vi "XY Sample Stage.vi"(7 "Calling VI Ref":refnum<vi>) -> ()   [LabVIEW 2020]
uses:
  <vilib>/Utility/miscctls.llb/LVPointTypeDef.ctl
  XY Sample Stage Controls/XY Sample Stage History Actions.ctl
  XY Sample Stage Controls/XY Sample Stage XY Settings.ctl
  Hardware Configuration/Hardware Configuration Controls/Device Function.ctl
  Hardware Configuration/Hardware Configuration Controls/Device Type.ctl
  Device Library/Stages/Stages Controls/Stage Actions.ctl
panel:
  in  "Main Tabs":enum32{"XY Control", "Settings"}(tab)
  in  "Remove Current":bool
  in  "Update Current":bool
  in  "Up":bool
  in  "Halt":bool
  in  "Down":bool
  in  "Left":bool
  in  "Right":bool
  in  "Home":bool
  in  "Mark Point":bool
  in  "Clear Points":bool
  in  "Marked Positions":i32(listbox)
  out "Position History":cluster{dbl[], dbl[]}[](graph)
  in  "X Position (µm)":dbl format="%#.6f"
  in  "Y Position (µm)":dbl format="%#.6f"
  in  "Step Size (µm)":dbl format="%#.3g"
  in  "Step 1":bool
  in  "Step 2":bool
  in  "Step 3":bool
  in  "Step 4":bool
  in  "Step 5":bool
  in  "Step 6":bool
  in  "Step 7":bool
  in  "Step 8":bool
  in  "Reset Location History":bool
  in  "Active Stage":i32(ring) items=["ASI-Stage-Sample XY-COM4", "Prior-Stage-Sample Z-0.1", "Thorlabs-Stage-Adj Cavity-65864035"]
  in  "Apply Offset":bool
  in  "Flip X and Y":bool
  in  "Invert X":bool
  in  "Invert Y":bool
  in  "Save XY Config":bool
  in  "Velocity":dbl=0.17 min=0.0 max=10000.0 format="%#.6f"
  in  "X Offset":dbl min=-10000.0 max=10000.0 format="%#.6f"
  in  "Y Offset":dbl min=-10000.0 max=10000.0 format="%#.6f"
  in  "Quit":bool
  # "Preset Step Sizes"
  # "Apply Offset to Marked Positions"
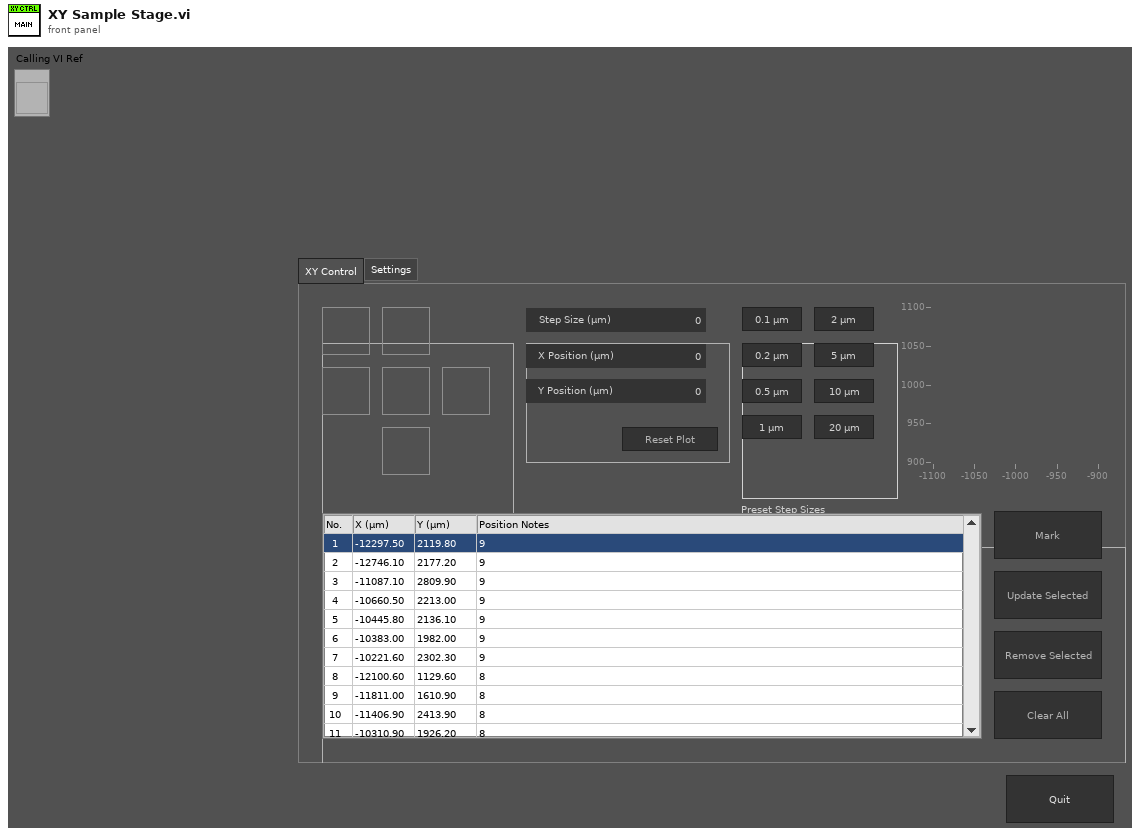
[diagram p1: front panel]
types:
  T1 = typedef "XY Sample Stage XY Settings.ctl" = cluster{"Flip X and Y":bool, "Invert X":bool, "Invert Y":bool}
  T2 = typedef "XY Sample Stage History Actions.ctl" = enum16{"Reset", "Write", "Read", "Set Zero", "Update", "Remove"}
  T3 = enum16{"Always On", "Always Off", "Off While Running"}
  T4 = typedef "LVPointTypeDef.ctl" = cluster{"Horizontal":i16, "Vertical":i16}
  T5 = typedef "LVRectTypeDef.ctl" = cluster{"Left":i16, "Top":i16, "Right":i16, "Bottom":i16}
  T6 = typedef "LVBoundsTypeDef.ctl" = cluster{"Width":u32, "Height":u32}
  T7 = typedef "Stage Actions.ctl" = enum16{"Get Position", "MVR", "MOVE", "HALT", "ONTARGET", "ERROR", "REFERENCE", "INIT", "VELOCITY", "STATUS", "EXIT", "HOME", "ZEROPOS", "NANOPOS", "ANALOG", "QUIT"}
  T8 = typedef "Device Type.ctl" = enum16{"AOTF", "Camera", "Deformable Mirror", "Laser", "Microscope Base", "Shutter", "Stage", "Waveform", "FPGA", "Email", "Filter Wheel", "Spinning Disk"}
  T9 = typedef "Device Function.ctl" = enum16{"Primary", "Secondary", "Overview", "Wide Field Drift Correction", "642 nm Excitation", "560 nm Excitation", "940 nm Excitation", "546 nm Excitation", "488 nm Excitation", "405 nm Excitation", "Objective Drift Correction", "4Pi Objective Lock", "Objective XY", "Objective Z", "Sample XY", "Sample Coarse Z", "Sample Z", "4Pi Lower", "4Pi Upper", "Mojo", "Adj Cavity", "Line Scanning", "Alert"}
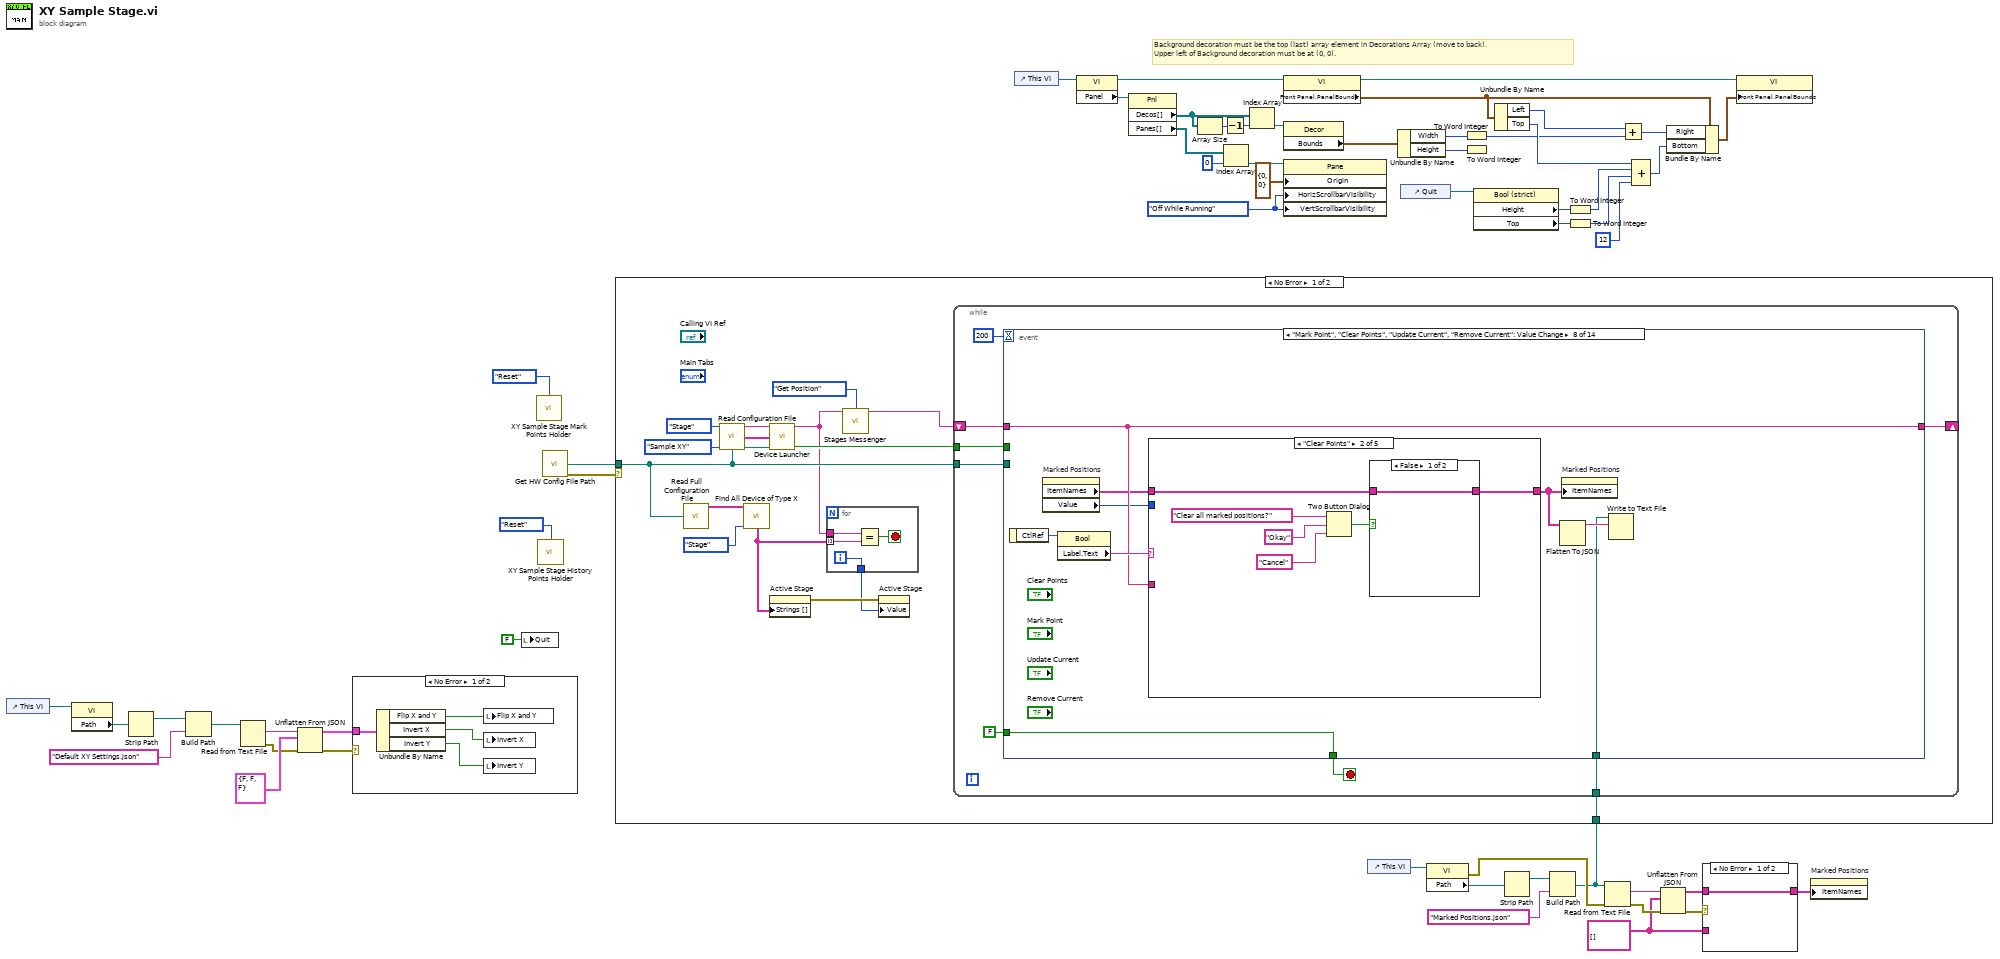
[diagram p0: block diagram]
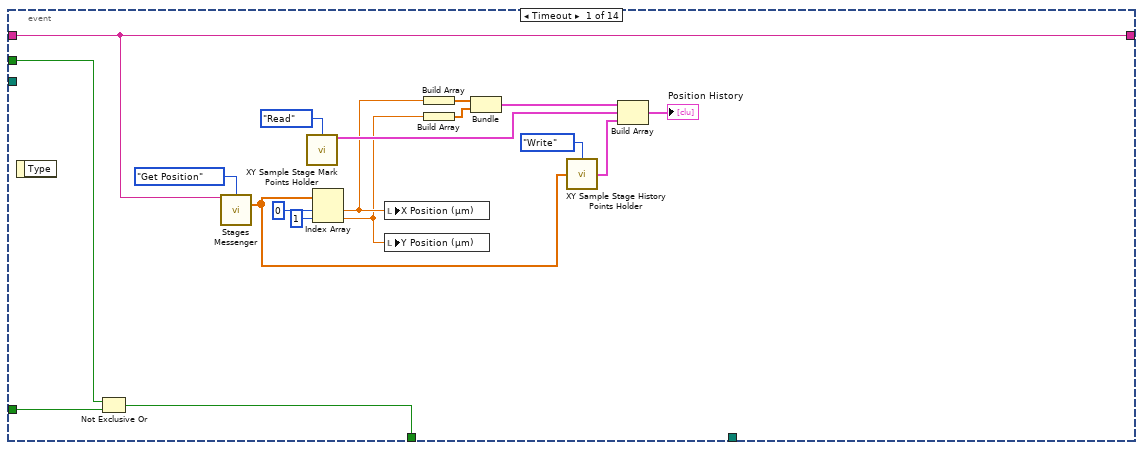
[diagram p4: hidden frame]
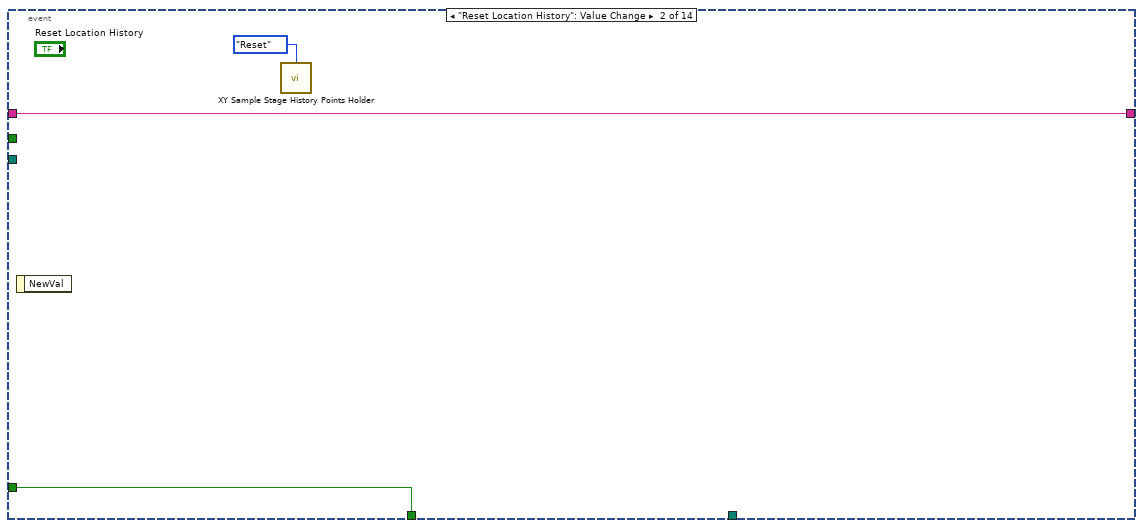
[diagram p5: hidden frame]
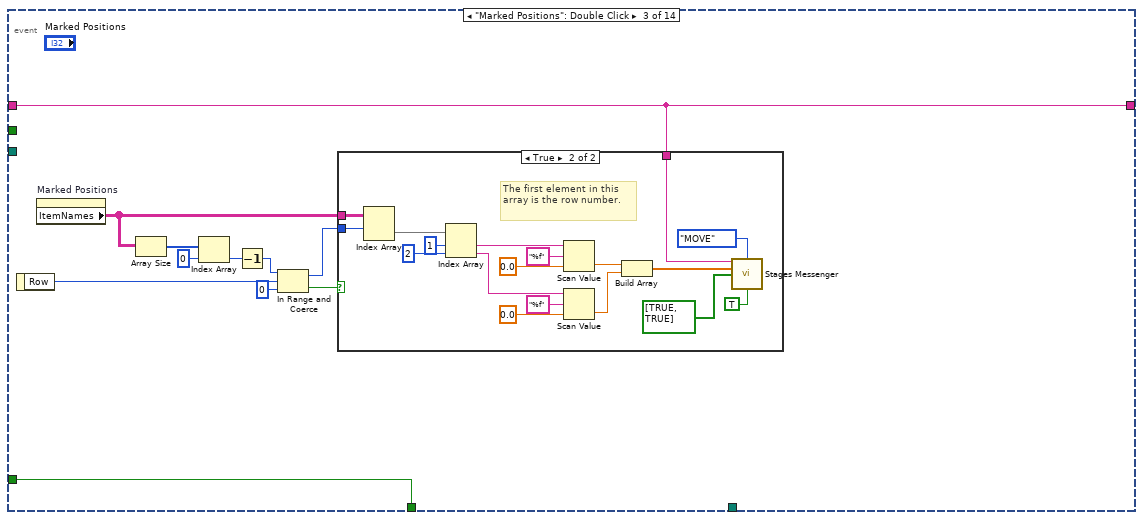
[diagram p6: hidden frame]
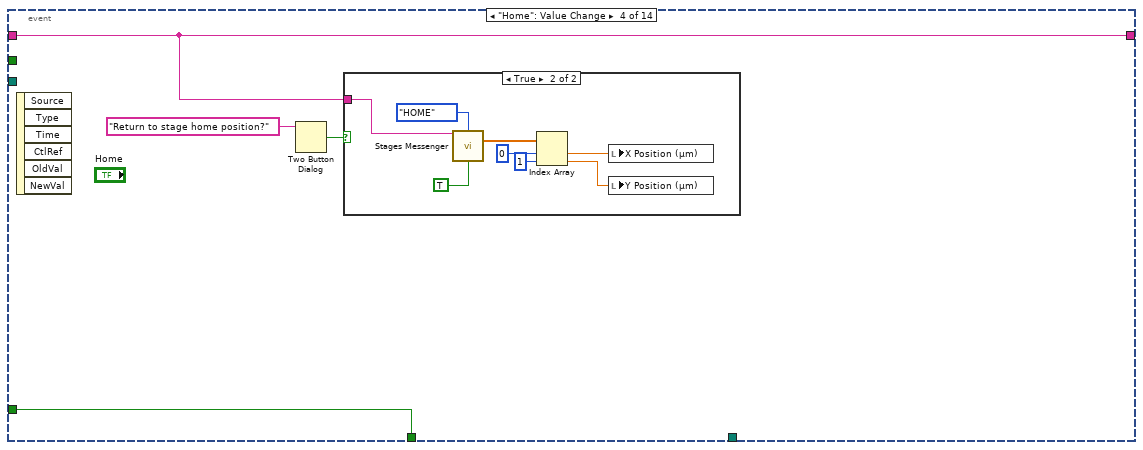
[diagram p8: hidden frame]
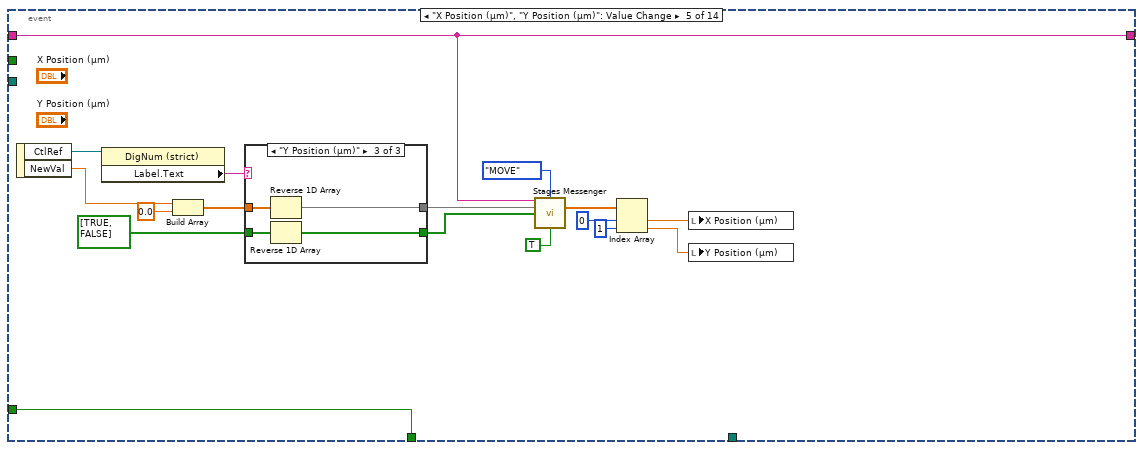
[diagram p10: hidden frame]
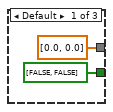
[diagram p11: hidden frame]
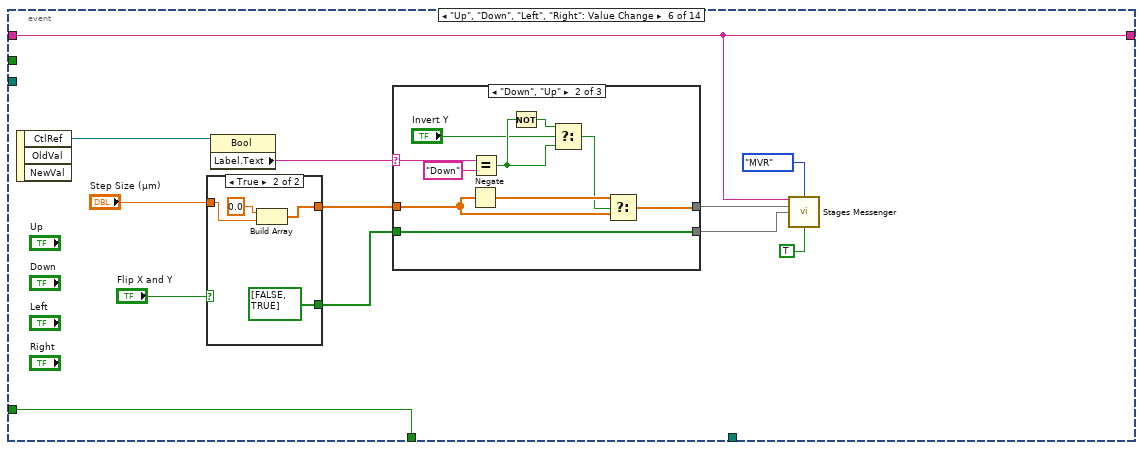
[diagram p13: hidden frame]
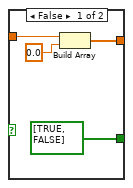
[diagram p14: hidden frame]
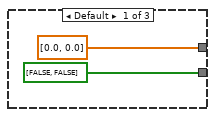
[diagram p15: hidden frame]
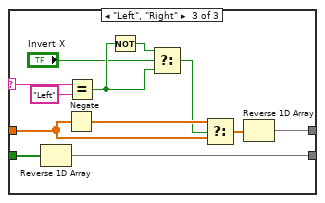
[diagram p16: hidden frame]
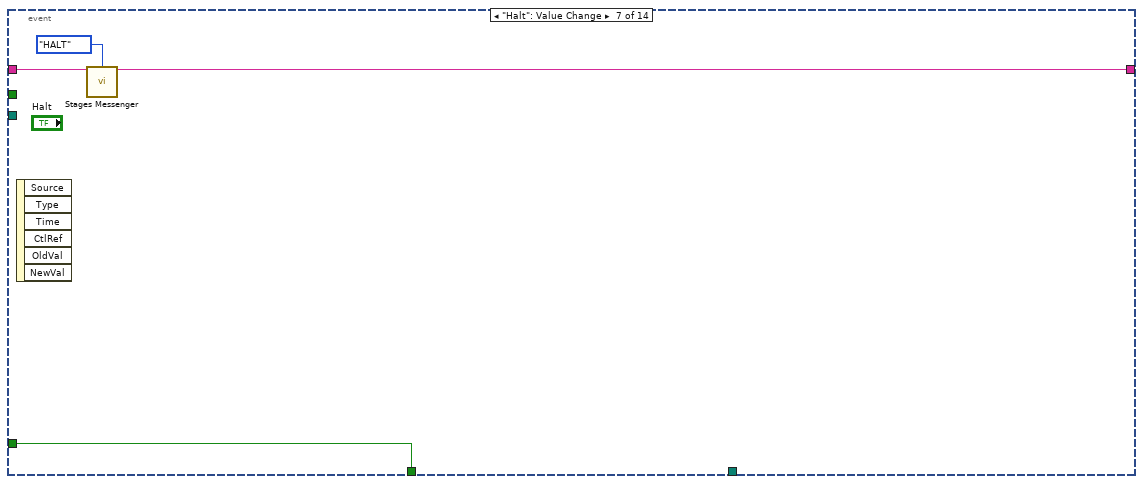
[diagram p17: hidden frame]
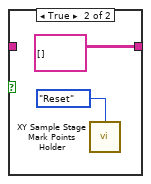
[diagram p19: hidden frame]
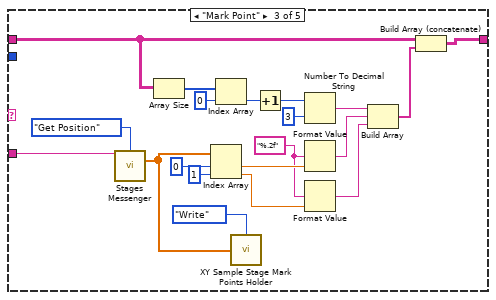
[diagram p20: hidden frame]
diagram:
  w2 = string[][] [] ("Item Names")
  w39 = T3."Off While Running" ("Vertical Scrollbar Visibility")
  # "Background decoration must be the top (last) array element in Decorations Array (move to back).\nUpper left of Background decoration must be at (0, 0)."
  n1 = control-ref of="This VI"() -> (w19:refnum<vi>)
  n2 = property class="VI"(reference=w19) -> ("Path"=w20:path)  [unwired: 1 in, 2 out]
  n3 = Strip Path(path=w20) -> (stripped path=w21:path)  [unwired: 1 out]
  n4 = Build Path(base path=w21, name or relative path="Default XY Settings.json") -> (appended path=w18:path)
  n5 = Read from Text File(file (use dialog)=w18) -> (text=w17:string, error out=w15:errorcluster)  [unwired: 3 in, 2 out]
  n6 = Unflatten From JSON(JSON string=w17, type and defaults=T1 {"Flip X and Y"=FALSE, "Invert X"=FALSE, "Invert Y"=FALSE} ("XY Flip Defaults"), error in (no error)=w15) -> (value=w13:T1, error out=w14:errorcluster)  [unwired: 4 in]
  n7 = case shown="No Error" w14 {
    tunnel: w13 -> [w60 _]
    frame No Error {
      n8 = Unbundle By Name(w60) -> ("Flip X and Y"=w59:bool, "Invert X"=w58:bool, "Invert Y"=w57:bool)
      n9 = local write "Flip X and Y"(w59) -> ()
      n10 = local write "Invert X"(w58) -> ()
      n11 = local write "Invert Y"(w57) -> ()
    }
    frame Error {
    }
  }
  n12 = local write "Quit"(FALSE ("Quit")) -> ()
  n13 = call "XY Sample Stage Mark Points Holder.vi"("Actions"=XY_Sample_Stage_History_Actions."Reset") -> ()  [unwired: 14 in, 1 out]
  n14 = call "XY Sample Stage History Points Holder.vi"("Actions"=XY_Sample_Stage_History_Actions."Reset") -> ()  [unwired: 14 in, 1 out]
  n15 = call "Get HW Config File Path.vi"() -> ("File Path"=w25:path, "Error"=w26:errorcluster)  [unwired: 14 in]
  n16 = control-ref of="This VI"() -> (w31:refnum<vi>)
  n17 = property class="VI"(reference=w31) -> (reference out=w40:refnum<vi>, "Panel"=w32:refnum<vi>)  [unwired: 1 in, 1 out]
  n18 = property class="Pnl"(reference=w32) -> ("Decos[]"=w30:refnum<vi>[], "Panes[]"=w36:refnum<vi>[])  [unwired: 1 in, 2 out]
  n19 = Array Size(array=w30) -> (size(s)=w28:i32)
  n20 = Decrement(x=w28) -> (x-1=w29:i32)
  n21 = Index Array(array=w36, index=0) -> (element=w35:refnum<vi>)
  n22 = Index Array(array=w30, index=w29) -> (element=w38:refnum<vi>)
  n23 = property class="VI"(reference=w40) -> (reference out=w42:refnum<vi>, "Front Panel.PanelBounds"=w43:T5)  [unwired: 1 in, 1 out]
  n24 = property class="Decor"(reference=w38) -> ("Bounds"=w41:T6)  [unwired: 1 in, 2 out]
  n25 = property class="Pane"(reference=w35, "Origin"=T4 {"Horizontal"=0, "Vertical"=0}, "HorizScrollbarVisibility"=w39, "VertScrollbarVisibility"=w39) -> ()  [unwired: 1 in, 2 out]
  n26 = control-ref of="This VI"() -> (w12:refnum<vi>)
  n27 = Unbundle By Name(w41) -> ("Width"=w46:u32, "Height"=w49:u32)
  n28 = control-ref of="Quit"() -> (w33:refnum<vi>)
  n29 = property class="VI"(reference=w12) -> (error out=w7:errorcluster, "Path"=w11:path)  [unwired: 1 in, 1 out]
  n30 = To Word Integer(number=w46) -> (16bit integer=w48:i16)
  n31 = To Word Integer(number=w49) -> ()  [unwired: 1 out]
  n32 = property class="Bool (strict)"(reference=w33) -> ("Height"=w51:u32, "Top"=w52:i32)  [unwired: 1 in, 2 out]
  n33 = Unbundle By Name(w43) -> ("Left"=w45:i16, "Top"=w56:i16)
  n34 = Strip Path(path=w11) -> (stripped path=w10:path)  [unwired: 1 out]
  n35 = Build Path(base path=w10, name or relative path="Marked Positions.json") -> (appended path=w1:path)
  n36 = case shown="No Error" w26 {
    tunnel: w25 -> [w65 _]
    tunnel: w1 -> [w61 _]
    frame No Error {
      n37 = call "Read Full Configuration File.vi"("Config File Path"=w65) -> ("Unique Notifier Names"=w70:string[])  [unwired: 11 in, 3 out]
      n38 = call "Read Configuration File.vi"("Device Type"=Device_Type."Stage", "Device Function"=Device_Function."Sample XY", "Config File Path"=w65) -> ("Unique Notifier Name"=w76:string, "Device Ports/IDs/Channels"=w74:string[], "Device Engine Path"=w75:path)  [unwired: 9 in, 1 out]
      n39 = call "Find All Device of Type X.vi"("Unique Notifier Names"=w70, "Device Type"=Device_Type."Stage") -> ("All Devices"=w68:string[])  [unwired: 12 in, 1 out]
      n40 = call "Device Launcher.vi"("Notifier Name"=w76, "Device Ports/IDs/Channels"=w74, "Device Engine Path"=w75) -> ("Notifier Name"=w63:string, "Running?"=w71:bool)  [unwired: 11 in]
      n41 = property on="Active Stage" class="Ring (strict)"("Strings []"=w68) -> (error out=w67:errorcluster)  [unwired: 2 in, 1 out]
      n42 = for {
        tunnel: w68 -> [w79] mode=indexing
        tunnel: w63 -> [w80]
        tunnel: [w77] -> w66
        i -> [w77]
        stop <- w78 stop-if-true
        n43 = Equal?(x=w80, y=w79) -> (x = y?=w78:bool)
      }
      n44 = call "Stages Messenger.vi"("Stage Notifier Name"=w63, "Actions"=Stage_Actions."Get Position") -> ("Stage Notifier Name (Dup)"=w62:string)  [unwired: 10 in, 3 out]
      n45 = property on="Active Stage" class="Ring (strict)"(error in=w67, "Value"=w66) -> ()  [unwired: 1 in, 2 out]
      n46 = while {
        tunnel: w71 -> [w85]
        shift-right: [w83] -> _
        shift-left: w62 -> [w86]
        tunnel: w65 -> [w82]
        tunnel: w61 -> [w81]
        stop <- w88 stop-if-true
        n47 = event shown="[7] \"Mark Point\", \"Clear Points\", \"Update Current\", \"Remove Current\": Value Change" {
          selector: _ -> [_ _ _ _ _ _ _ _ _ _ _ _ _ _]
          dyn-events: _ -> [_ _ _ _ _ _ _ _ _ _ _ _ _ _]
          timeout: 200 -> [_ _ _ _ _ _ _ _ _ _ _ _ _ _]
          tunnel: [w92 w109 w120 w142 w167 w187 w222 w232 w300 w313 w325 w341 w378 TRUE ("NewVal")] -> w88
          tunnel: FALSE ("NewVal") -> [w93 w109 w120 w142 w167 w187 w222 w232 w300 w313 w325 w341 w378 _]
          tunnel: w86 -> [w91 w108 w119 w139 w151 w178 w221 w229 w299 w301 _ w336 w367 w388]
          tunnel: w85 -> [w94 _ _ _ _ _ _ _ _ _ _ _ _ _]
          tunnel: [w91 w108 w119 w139 w151 w178 w220 w229 w296 w301 w314 w336 w367 w388] -> w83
          tunnel: w82 -> [_ _ _ _ _ _ _ _ _ _ w323 _ _ _]
          tunnel: w81 -> [_ _ _ _ _ _ _ w226 _ _ _ _ _ _]
          event Timeout {
            n48 = event-data() -> ()  [unwired: 1 in, 1 out]
            n49 = Not Exclusive Or(1:w93, 2:w94) -> (0:w92:bool)
            n50 = call "Stages Messenger.vi"("Stage Notifier Name"=w91, "Actions"=Stage_Actions."Get Position") -> ("Positions"=w98:dbl[])  [unwired: 10 in, 3 out]
            n51 = call "XY Sample Stage Mark Points Holder.vi"("Actions"=XY_Sample_Stage_History_Actions."Read") -> ("Marked Points"=w95:cluster{dbl[], dbl[]})  [unwired: 14 in]
            n52 = Index Array(array=w98, index #1=0 ("index"), index #2=1 ("index")) -> (element #1=w90:dbl, element #2=w89:dbl)
            n53 = local write "X Position (µm)"(w90) -> ()
            n54 = local write "Y Position (µm)"(w89) -> ()
            n55 = Build Array(w90) -> (w103:dbl[])
            n56 = Build Array(w89) -> (w102:dbl[])
            n57 = Bundle(w103, w102) -> (w96:cluster{dbl[], dbl[]})  [unwired: 1 in]
            n58 = call "XY Sample Stage History Points Holder.vi"("Actions"=XY_Sample_Stage_History_Actions."Write", "(x, y) Points"=w98) -> ("History Points"=w101:cluster{dbl[], dbl[]})  [unwired: 13 in]
            n59 = Build Array(w96, w95, w101) -> (→"Position History":cluster{dbl[], dbl[]}[])
          }
          event "Reset Location History": Value Change {
            n60 = event-data() -> ()  [unwired: 1 in, 1 out]
            n61 = call "XY Sample Stage History Points Holder.vi"("Actions"=XY_Sample_Stage_History_Actions."Reset") -> ()  [unwired: 14 in, 1 out]
          }
          event "Marked Positions": Double Click {
            n62 = event-data() -> ("Row"=w117:i32)  [unwired: 1 in]
            n63 = property on="Marked Positions" class="MCListbox (strict)"() -> ("ItemNames"=w118:string[][])  [unwired: 2 in, 2 out]
            n64 = Array Size(array=w118) -> (size(s)=w115:i32[])
            n65 = Index Array(array=w115, index=0) -> (element=w113:i32)
            n66 = Decrement(x=w113) -> (x-1=w112:i32)
            n67 = In Range and Coerce(upper limit=w112, x=w117, lower limit=0) -> (coerced(x)=w111:i32, In Range?=w110:bool)
            n68 = case shown="True" w110 {
              tunnel: w119 -> [_ w124]
              tunnel: w118 -> [_ w122]
              tunnel: w111 -> [_ w121]
              frame False {
              }
              frame True {
                # "The first element in this array is the row number."
                n69 = Index Array(array=w122, index (row)=w121) -> (element=w133:string[])  [unwired: 1 in]
                n70 = Index Array(array=w133, index #1=1 ("index"), index #2=2 ("index")) -> (element #1=w128:string, element #2=w123:string)
                n71 = Scan Value(string=w128, format string="%f", default (0 dbl)=0.0) -> (value=w127:dbl)  [unwired: 1 out]
                n72 = Scan Value(string=w123, format string="%f", default (0 dbl)=0.0) -> (value=w126:dbl)  [unwired: 1 out]
                n73 = Build Array(w127, w126) -> (w125:dbl[])
                n74 = call "Stages Messenger.vi"("Stage Notifier Name"=w124, "Actions"=Stage_Actions."MOVE", "Setpoint"=w125, "Axis"=bool[] [TRUE, TRUE], "Exit While Busy?"=TRUE ("Wait for On Target? (F)")) -> ()  [unwired: 7 in, 4 out]
              }
            }
          }
          event "Home": Value Change {
            n75 = event-data() -> ()  [unwired: 1 in, 6 out]
            n76 = Two Button Dialog(message="Return to stage home position?") -> (T button?=w140:bool)  [unwired: 2 in]
            n77 = case shown="True" w140 {
              tunnel: w139 -> [_ w149]
              frame False {
              }
              frame True {
                n78 = call "Stages Messenger.vi"("Stage Notifier Name"=w149, "Actions"=Stage_Actions."HOME", "Exit While Busy?"=TRUE) -> ("Positions"=w144:dbl[])  [unwired: 9 in, 3 out]
                n79 = Index Array(array=w144, index #1=0 ("index"), index #2=1 ("index")) -> (element #1=w146:dbl, element #2=w145:dbl)
                n80 = local write "X Position (µm)"(w146) -> ()
                n81 = local write "Y Position (µm)"(w145) -> ()
              }
            }
          }
          event "X Position (µm)", "Y Position (µm)": Value Change {
            n82 = event-data() -> ("CtlRef"=w166:refnum<vi>, "NewVal"=w163:dbl)  [unwired: 1 in]
            n83 = property class="DigNum (strict)"(reference=w166) -> ("Label.Text"=w165:string)  [unwired: 1 in, 2 out]
            n84 = Build Array(w163, 0.0 ("element")) -> (w162:dbl[])
            n85 = case shown="\"Y Position (µm)\"" w165 {
              tunnel: w162 -> [_ w171 w175]
              tunnel: bool[] [TRUE, FALSE] -> [_ w170 w174]
              tunnel: [dbl[] [0.0, 0.0] w171 w173] -> w159
              tunnel: [bool[] [FALSE, FALSE] w170 w172] -> w158
              frame Default {
              }
              frame "X Position (µm)" {
              }
              frame "Y Position (µm)" {
                n86 = Reverse 1D Array(array=w175) -> (reversed array=w173:dbl[])
                n87 = Reverse 1D Array(array=w174) -> (reversed array=w172:bool[])
              }
            }
            n88 = call "Stages Messenger.vi"("Stage Notifier Name"=w151, "Actions"=Stage_Actions."MOVE", "Setpoint"=w159, "Axis"=w158, "Exit While Busy?"=TRUE ("Wait for On Target? (F)")) -> ("Positions"=w152:dbl[])  [unwired: 7 in, 3 out]
            n89 = Index Array(array=w152, index #1=0 ("index"), index #2=1 ("index")) -> (element #1=w154:dbl, element #2=w153:dbl)
            n90 = local write "X Position (µm)"(w154) -> ()
            n91 = local write "Y Position (µm)"(w153) -> ()
          }
          event "Up", "Down", "Left", "Right": Value Change {
            n92 = event-data() -> ("CtlRef"=w186:refnum<vi>)  [unwired: 1 in, 2 out]
            n93 = case shown="True" "Flip X and Y" {
              tunnel: [bool[] [TRUE, FALSE] bool[] [FALSE, TRUE]] -> w180
              tunnel: [w189 w194] -> w179
              tunnel: "Step Size (µm)" -> [w188 w193]
              frame False {
                n94 = Build Array(w188, 0.0 ("element")) -> (w189:dbl[])
              }
              frame True {
                n95 = Build Array(0.0 ("element"), w193) -> (w194:dbl[])
              }
            }
            n96 = property class="Bool"(reference=w186) -> ("Label.Text"=w185:string)  [unwired: 1 in, 2 out]
            n97 = case shown="\"Down\", \"Up\"" w185 {
              selector: w185 -> [_ w207 w217]
              tunnel: w179 -> [_ w204 w216]
              tunnel: w180 -> [_ w202 w214]
              tunnel: [dbl[] [0.0, 0.0] w203 w213] -> w182
              tunnel: [bool[] [FALSE, FALSE] w202 w212] -> w181
              frame Default {
              }
              frame "Down", "Up" {
                n98 = Negate(x=w204) -> (-x=w205:dbl[])
                n99 = Equal?(x=w207, y="Down") -> (x = y?=w201:bool)
                n100 = Not(x=w201) -> (.not. x?=w200:bool)
                n101 = Select(t=w200, s="Invert Y", f=w201) -> (s? t:f=w199:bool)
                n102 = Select(t=w205, s=w199, f=w204) -> (s? t:f=w203:dbl[])
              }
              frame "Left", "Right" {
                n103 = Reverse 1D Array(array=w214) -> (reversed array=w212:bool[])
                n104 = Negate(x=w216) -> (-x=w218:dbl[])
                n105 = Equal?(x=w217, y="Left") -> (x = y?=w210:bool)
                n106 = Not(x=w210) -> (.not. x?=w211:bool)
                n107 = Select(t=w211, s="Invert X", f=w210) -> (s? t:f=w209:bool)
                n108 = Select(t=w218, s=w209, f=w216) -> (s? t:f=w215:dbl[])
                n109 = Reverse 1D Array(array=w215) -> (reversed array=w213:dbl[])
              }
            }
            n110 = call "Stages Messenger.vi"("Stage Notifier Name"=w178, "Actions"=Stage_Actions."MVR", "Setpoint"=w182, "Axis"=w181, "Exit While Busy?"=TRUE ("Wait for On Target? (F)")) -> ()  [unwired: 7 in, 4 out]
          }
          event "Halt": Value Change {
            n111 = event-data() -> ()  [unwired: 1 in, 6 out]
            n112 = call "Stages Messenger.vi"("Stage Notifier Name"=w221, "Actions"=Stage_Actions."HALT") -> ("Stage Notifier Name (Dup)"=w220:string)  [unwired: 10 in, 3 out]
          }
          event "Mark Point", "Clear Points", "Update Current", "Remove Current": Value Change {
            n113 = event-data() -> ("CtlRef"=w231:refnum<vi>)  [unwired: 1 in]
            n114 = property on="Marked Positions" class="MCListbox (strict)"() -> ("ItemNames"=w225:string[][], "Value"=w224:i32)  [unwired: 2 in, 2 out]
            n115 = property class="Bool"(reference=w231) -> ("Label.Text"=w230:string)  [unwired: 1 in, 2 out]
            n116 = case shown="\"Clear Points\"" w230 {
              tunnel: [w233 w239 w244 w267 w281] -> w227
              tunnel: w229 -> [_ _ w245 w268 _]
              tunnel: w225 -> [w233 w238 w243 w265 w290]
              tunnel: w224 -> [_ _ _ w264 w289]
              frame Default {
              }
              frame "Clear Points" {
                n117 = Two Button Dialog(message="Clear all marked positions?", 1:"Cancel" ("F button name (\"Cancel\")"), 2:"Okay" ("T button name (\"OK\")")) -> (T button?=w234:bool)
                n118 = case shown="False" w234 {
                  tunnel: [w240 string[][] []] -> w239
                  tunnel: w238 -> [w240 _]
                  frame False {
                  }
                  frame True {
                    n119 = call "XY Sample Stage Mark Points Holder.vi"("Actions"=XY_Sample_Stage_History_Actions."Reset") -> ()  [unwired: 14 in, 1 out]
                  }
                }
              }
              frame "Mark Point" {
                w257 = "%.2f" ("format string")
                n120 = call "Stages Messenger.vi"("Stage Notifier Name"=w245, "Actions"=Stage_Actions."Get Position") -> ("Positions"=w247:dbl[])  [unwired: 10 in, 3 out]
                n121 = Array Size(array=w243) -> (size(s)=w254:i32[])
                n122 = Index Array(array=w247, index #1=0 ("index"), index #2=1 ("index")) -> (element #1=w259:dbl, element #2=w258:dbl)
                n123 = Index Array(array=w254, index=0) -> (element=w252:i32)
                n124 = call "XY Sample Stage Mark Points Holder.vi"("Actions"=XY_Sample_Stage_History_Actions."Write", "(X, Y) Points"=w247) -> ()  [unwired: 13 in, 1 out]
                n125 = Increment(x=w252) -> (x+1=w256:i32)
                n126 = Number To Decimal String(number=w256, width (-)=i16 3) -> (decimal integer string=w251:string)
                n127 = Format Value(format string=w257, value (0)=w259) -> (output string=w249:string)  [unwired: 1 in]
                n128 = Format Value(format string=w257, value (0)=w258) -> (output string=w250:string)  [unwired: 1 in]
                n129 = Build Array(w251, w249, w250) -> (w248:string[])
                n130 = Build Array (concatenate)(w243, w248) -> (w244:string[][])
              }
              frame "Update Current" {
                w275 = "%.2f" ("format string")
                n131 = call "Stages Messenger.vi"("Stage Notifier Name"=w268, "Actions"=Stage_Actions."Get Position") -> ("Positions"=w270:dbl[])  [unwired: 10 in, 3 out]
                n132 = Index Array(array=w270, index #1=0 ("index"), index #2=1 ("index")) -> (element #1=w277:dbl, element #2=w276:dbl)
                n133 = Increment(x=w264) -> (x+1=w263:i32)
                n134 = call "XY Sample Stage Mark Points Holder.vi"("Index"=w264, "Actions"=XY_Sample_Stage_History_Actions."Update", "(X, Y) Points"=w270) -> ()  [unwired: 12 in, 1 out]
                n135 = Number To Decimal String(number=w263, width (-)=i16 3) -> (decimal integer string=w273:string)
                n136 = Format Value(format string=w275, value (0)=w277) -> (output string=w271:string)  [unwired: 1 in]
                n137 = Format Value(format string=w275, value (0)=w276) -> (output string=w272:string)  [unwired: 1 in]
                n138 = Build Array(w273, w271, w272) -> (w266:string[])
                n139 = Replace Array Subset(array=w265, new element=w266, index (row)=w264) -> (w267:string[][])  [unwired: 1 in]
              }
              frame "Remove Current" {
                n140 = Delete From Array(array=w290, length=1, index (row)=w289) -> (array with subset deleted=w284:string[][])  [unwired: 1 in, 1 out]
                n141 = call "XY Sample Stage Mark Points Holder.vi"("Index"=w289, "Actions"=XY_Sample_Stage_History_Actions."Remove") -> ()  [unwired: 13 in, 1 out]
                n142 = Array Size(array=w284) -> (size(s)=w287:i32[])
                n143 = Index Array(array=w287, index=0) -> (element=w285:i32)
                n144 = for {
                  N: w285 -> [_]
                  tunnel: [w292] -> w282 mode=indexing
                  i -> [w295]
                  n145 = Increment(x=w295) -> (x+1=w293:i32)
                  n146 = Number To Decimal String(number=w293, width (-)=i16 3) -> (decimal integer string=w292:string)
                }
                n147 = Replace Array Subset(array=w284, new element=w282, index (col)=0 ("disabled index (col)")) -> (w281:string[][])  [unwired: 1 in]
              }
            }
            n148 = Flatten To JSON(anything=w227) -> (JSON string=w228:string)  [unwired: 2 in, 1 out]
            n149 = property on="Marked Positions" class="MCListbox (strict)"("ItemNames"=w227) -> ()  [unwired: 2 in, 2 out]
            n150 = Write to Text File(file (use dialog)=w226, text=w228) -> ()  [unwired: 2 in, 3 out]
          }
          event "Velocity": Value Change {
            n151 = event-data() -> ("NewVal"=w297:dbl)  [unwired: 1 in]
            n152 = call "Stages Messenger.vi"("Stage Notifier Name"=w299, "Actions"=Stage_Actions."VELOCITY", "Velocity"=w297) -> ("Stage Notifier Name (Dup)"=w296:string)  [unwired: 9 in, 3 out]
          }
          event "Save XY Config": Value Change {
            n153 = event-data() -> ()  [unwired: 1 in, 1 out]
            n154 = control-ref of="This VI"() -> (w312:refnum<vi>)
            n155 = local read "Flip X and Y"() -> (w307:bool)
            n156 = local read "Invert X"() -> (w306:bool)
            n157 = local read "Invert Y"() -> (w305:bool)
            n158 = property class="VI"(reference=w312) -> ("Path"=w311:path)  [unwired: 1 in, 2 out]
            n159 = Bundle By Name(cluster=T1 {"Flip X and Y"=FALSE, "Invert X"=TRUE, "Invert Y"=TRUE} ("XY Flip Defaults"), "Flip X and Y"=w307, "Invert X"=w306, "Invert Y"=w305) -> (w304:T1)
            n160 = Strip Path(path=w311) -> (stripped path=w310:path)  [unwired: 1 out]
            n161 = Build Path(base path=w310, name or relative path="Default XY Settings.json") -> (appended path=w303:path)
            n162 = Flatten To JSON(anything=w304) -> (JSON string=w302:string)  [unwired: 2 in, 1 out]
            n163 = Write to Text File(file (use dialog)=w303, text=w302) -> ()  [unwired: 2 in, 3 out]
          }
          event "Active Stage": Value Change {
            n164 = event-data() -> ("CtlRef"=w324:refnum<vi>)  [unwired: 1 in]
            n165 = property class="Ring (strict)"(reference=w324) -> ("RingText.Text"=w322:string)  [unwired: 1 in, 2 out]
            n166 = call "Read Full Configuration File.vi"("Config File Path"=w323) -> ("Unique Notifier Names"=w321:string[], "Device Port/ID/Channel Info"=w320:string[][], "Device Engine Paths"=w319:path[])  [unwired: 11 in, 1 out]
            n167 = for {
              tunnel: w322 -> [w328]
              tunnel: w321 -> [w329] mode=indexing
              tunnel: [w326] -> w318
              i -> [w326]
              stop <- w327 stop-if-true
              n168 = Equal?(x=w329, y=w328) -> (x = y?=w327:bool)
            }
            n169 = Index Array(array=w321, index=w318) -> (element=w317:string)
            n170 = Index Array(array=w320, index (row)=w318) -> (element=w316:string[])  [unwired: 1 in]
            n171 = Index Array(array=w319, index=w318) -> (element=w315:path)
            n172 = call "Device Launcher.vi"("Notifier Name"=w317, "Device Ports/IDs/Channels"=w316, "Device Engine Path"=w315) -> ("Notifier Name"=w314:string)  [unwired: 11 in, 1 out]
          }
          event "Apply Offset": Value Change {
            n173 = event-data() -> ()  [unwired: 1 in, 1 out]
            n174 = property on="Marked Positions" class="MCListbox (strict)"() -> ("ItemNames"=w340:string[][])  [unwired: 2 in, 2 out]
            n175 = Array Size(array=w340) -> (size(s)=w339:i32[])
            n176 = Index Array(array=w339, index=0) -> (element=w337:i32)
            n177 = for {
              N: w337 -> [_]
              tunnel: w340 -> [w366]
              tunnel: [w353] -> w335 mode=indexing
              tunnel: [w349] -> w334 mode=indexing
              tunnel: [w348] -> w333 mode=indexing
              tunnel: [w342] -> w330 mode=indexing
              i -> [w354]
              w352 = "%.2f" ("format string")
              n178 = Index Array(array=w366, index (row)=w354) -> (element=w363:string[])  [unwired: 1 in]
              n179 = Increment(x=w354) -> (x+1=w355:i32)
              n180 = Index Array(array=w363, index #1=1 ("index"), index #2=2 ("index"), index #3=3 ("index")) -> (element #1=w358:string, element #2=w357:string, element #3=w342:string)
              n181 = Number To Decimal String(number=w355, width (-)=i16 3) -> (decimal integer string=w353:string)
              n182 = Scan Value(string=w358, format string="%f", default (0 dbl)=0.0) -> (value=w347:dbl)  [unwired: 1 out]
              n183 = Scan Value(string=w357, format string="%f", default (0 dbl)=0.0) -> (value=w346:dbl)  [unwired: 1 out]
              n184 = Add(x="X Offset", y=w347) -> (x+y=w351:dbl)
              n185 = Add(x=w346, y="Y Offset") -> (x+y=w350:dbl)
              n186 = Format Value(format string=w352, value (0)=w351) -> (output string=w349:string)  [unwired: 1 in]
              n187 = Format Value(format string=w352, value (0)=w350) -> (output string=w348:string)  [unwired: 1 in]
            }
            n188 = Build Array(w335, w334, w333, w330) -> (w332:string[][])
            n189 = Transpose 2D Array(2D array=w332) -> (transposed array=w331:string[][])
            n190 = property on="Marked Positions" class="MCListbox (strict)"("ItemNames"=w331) -> ()  [unwired: 2 in, 2 out]
          }
          event "Step 1", "Step 2", "Step 3", "Step 4", "Step 5", "Step 6", "Step 7", "Step 8": Value Change {
            n191 = event-data() -> ("CtlRef"=w369:refnum<vi>)  [unwired: 1 in]
            n192 = property class="Bool"(reference=w369) -> ("Label.Text"=w377:string)  [unwired: 1 in, 2 out]
            n193 = Reverse String(1:w377) -> (0:w376:string)
            n194 = String Subset(string=w376, offset (0)=0, length (rest)=1 ("length (rest)")) -> (substring=w373:string)
            n195 = Scan From String(format string="%d", input string=w373, default 1=-1 ("default value 1")) -> (output 1=w370:i32)  [unwired: 2 in, 3 out]
            n196 = case shown="0, Default" w370 {
              tunnel: [0.1 0.1 0.2 0.5 1.0 2.0 5.0 10.0 20.0] -> w368
              frame 0, Default {
              }
              frame 1 {
              }
              frame 2 {
              }
              frame 3 {
              }
              frame 4 {
              }
              frame 5 {
              }
              frame 6 {
              }
              frame 7 {
              }
              frame 8 {
              }
            }
            n197 = local write "Step Size (µm)"(w368) -> ()
          }
          event "Quit": Value Change {
            n198 = event-data() -> ()  [unwired: 1 in, 6 out]
          }
        }
      }
    }
    frame Error {
      n199 = control-ref of="This VI"() -> (w395:refnum<vi>)
      n200 = property class="VI"(reference=w395) -> ("Name"=w393:string)  [unwired: 1 in, 2 out]
      n201 = Concatenate Strings("Error in ", w393, "\r", "No Config File") -> (w390:string)
      n202 = One Button Dialog(message=w390) -> ()  [unwired: 1 in, 1 out]
    }
  }
  n203 = To Word Integer(number=w51) -> (16bit integer=w54:i16)
  n204 = To Word Integer(number=w52) -> (16bit integer=w55:i16)
  n205 = Read from Text File(file (use dialog)=w1, error in=w7) -> (text=w8:string, error out=w6:errorcluster)  [unwired: 2 in, 2 out]
  n206 = Add(x=w45, y=w48) -> (x+y=w47:i16)
  n207 = Compound Arithmetic op=ADD(w56, w54, w55, i16 12 ("y")) -> (w50:i16)
  n208 = Unflatten From JSON(JSON string=w8, type and defaults=w2, error in (no error)=w6) -> (value=w4:string[][], error out=w5:errorcluster)  [unwired: 4 in]
  n209 = Bundle By Name(cluster=w43, "Right"=w47, "Bottom"=w50) -> (w44:T5)
  n210 = case shown="No Error" w5 {
    tunnel: w4 -> [w396 _]
    tunnel: [w396 w397] -> w3
    tunnel: w2 -> [_ w397]
    frame No Error {
    }
    frame Error {
    }
  }
  n211 = property class="VI"(reference=w42, "Front Panel.PanelBounds"=w44) -> ()  [unwired: 1 in, 2 out]
  n212 = property on="Marked Positions" class="MCListbox (strict)"("ItemNames"=w3) -> ()  [unwired: 2 in, 2 out]
